vi "read_params.vi"(8 "error in (no error)":errorcluster, 11 "BayesianRidge in":refnum<class "BayesianRidge.lvclass">) -> (0 "error out":errorcluster, 2 "params":T1={"n_iter"=300.0, "tol"=0.001, "alpha_1"=1e-06, "alpha_2"=1e-06, "lambda_1"=1e-06, "lambda_2"=1e-06, "alpha_init"={"alpha_init_type"="None", "alpha_init_float"=0.0}, "lambda_init"={"lambda_init_type"="None", "lambda_init_float"=0.0}, "compute_score"=FALSE, "fit_intercept"=TRUE, "normalize"=FALSE, "copy_X"=TRUE, "verbose"=FALSE}, 3 "BayesianRidge out":refnum<class "BayesianRidge.lvclass">)   [LabVIEW 2020, in "BayesianRidge.lvclass"]
uses:
  BayesianRidge.lvclass
  Controls/bayesian_ridge_params.ctl
  BayesianRidge.lvclass/BayesianRidge.ctl
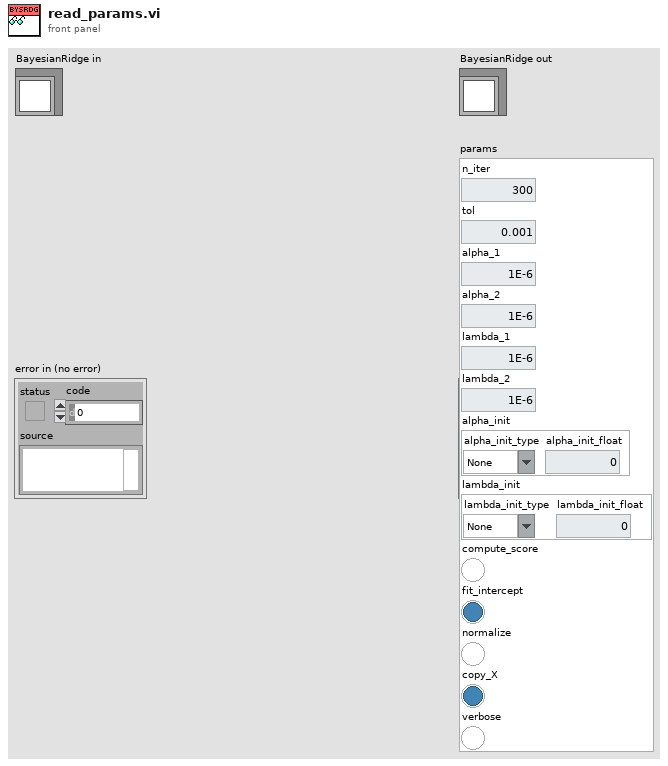
[diagram p1: front panel]
types:
  T1 = typedef "bayesian_ridge_params.ctl" = cluster{"n_iter":dbl, "tol":dbl, "alpha_1":dbl, "alpha_2":dbl, "lambda_1":dbl, "lambda_2":dbl, "alpha_init":cluster{"alpha_init_type":string, "alpha_init_float":dbl}, "lambda_init":cluster{"lambda_init_type":string, "lambda_init_float":dbl}, "compute_score":bool, "fit_intercept":bool, "normalize":bool, "copy_X":bool, "verbose":bool}
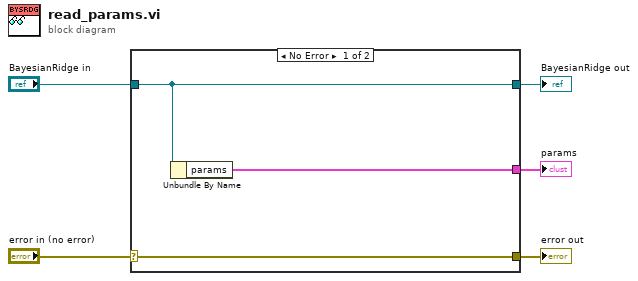
[diagram p0: block diagram]
diagram:
  n1 = case shown="No Error" "error in (no error)" {
    selector: "error in (no error)" -> [w8 w9]
    tunnel: [w8 w9] -> w4
    tunnel: [w7 w10] -> w2
    tunnel: "BayesianRidge in" -> [w7 w10]
    tunnel: [w6 _] -> w1
    frame No Error {
      n2 = Unbundle By Name(w7) -> ("params"=w6:T1)
    }
    frame Error {
    }
  }
  "error out" <- w4
  "BayesianRidge out" <- w2
  "params" <- w1
